vi "addSkipped.vi"(8 "error in (no error)":errorcluster, 10 "test":refnum<class>, 11 "TestResult in":refnum<class "TestResult.lvclass">) -> (0 "error out":errorcluster, 3 "TestResult out":refnum<class "TestResult.lvclass">)   [LabVIEW 2019, in "TestResult.lvclass"]
uses:
  TestResult.lvclass
  resultStatus--enum.ctl
  resultStatusChanged--Cluster.ctl
  TestResult.lvclass/TestResult.ctl
panel:
  # "JKI VI Tester for LabVIEW\nhttp://jkisoft.com/vi-tester\nCopyright (C) 2007-2009, JKI <info@jkisoft.com>\nALL RIGHTS RESERVED"
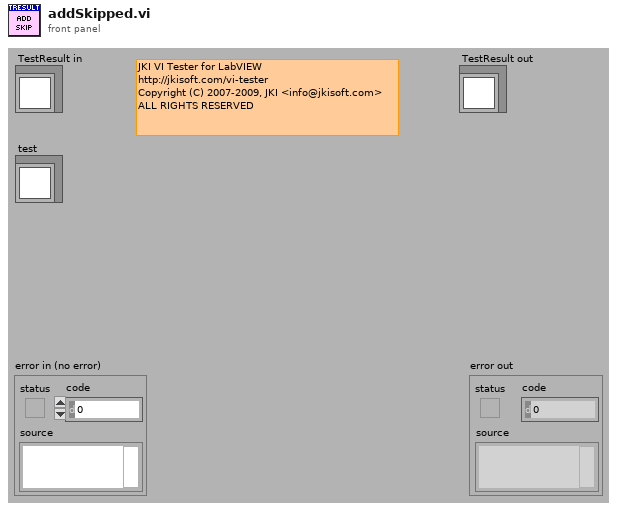
[diagram p1: front panel]
types:
  T1 = typedef "TestResult.lvclass/resultStatusChanged--Cluster.ctl" = cluster{"test":refnum<class>, "resultStatus":T2, "TestResult":refnum<class>, "test error":errorcluster, "execution time (sec)":dbl}
  T2 = typedef "TestResult.lvclass/resultStatus--enum.ctl" = enum16{"testPass", "testFailure", "testError", "testSkipped"}
  T3 = cluster{"test":refnum<class>, "skip error":errorcluster}
  T4 = typedef "TestResult.lvclass/skipped.ctl" = T5[]
  T5 = typedef "TestResult.lvclass/skip.ctl" = cluster{"test":refnum<class>, "error":errorcluster}
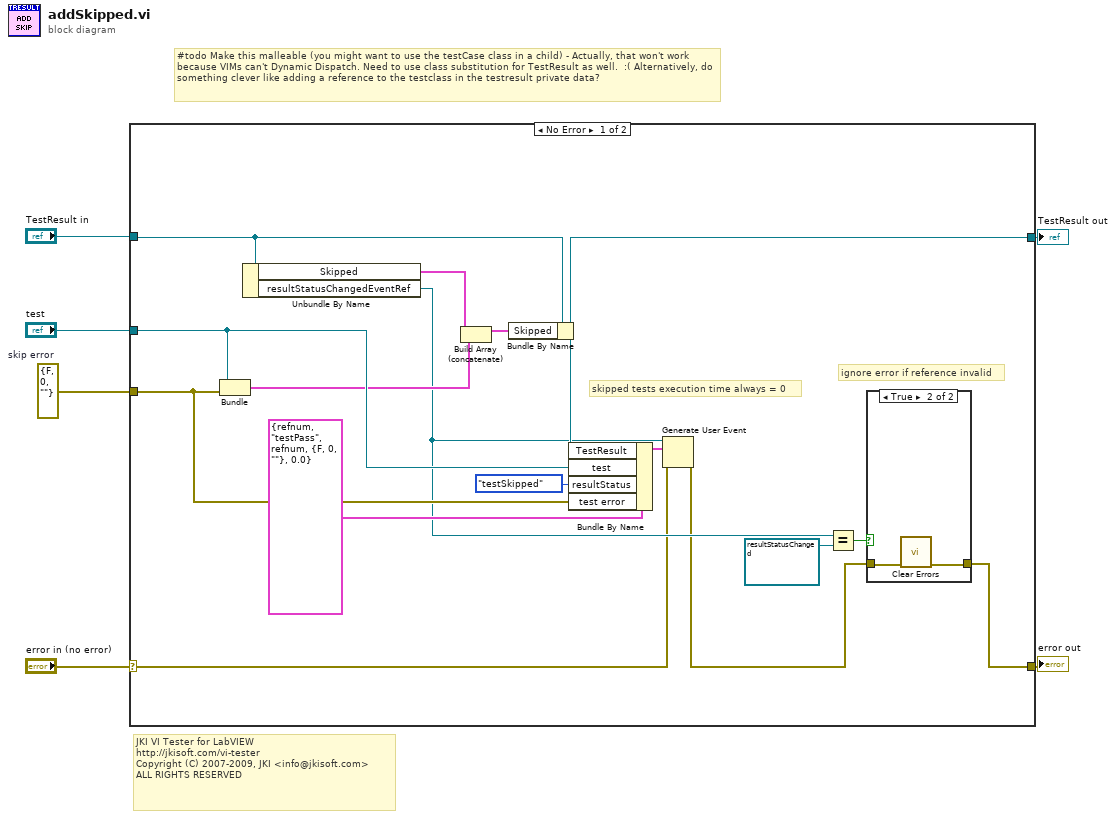
[diagram p0: block diagram]
diagram:
  w1 = errorcluster {"status"=FALSE, "code"=0, "source"=""}  # skip error
  # "#todo Make this malleable (you might want to use the testCase class in a child) - Actually, that won't work because VIMs can't Dynamic Dispatch. Need to use class substitution for TestResult as well.  :( Alternatively, do something clever like adding a reference to the testclass in the testresult private data?"
  # "JKI VI Tester for LabVIEW\nhttp://jkisoft.com/vi-tester\nCopyright (C) 2007-2009, JKI <info@jkisoft.com>\nALL RIGHTS RESERVED"
  n1 = case shown="No Error" "error in (no error)" {
    selector: "error in (no error)" -> [w9 w27]
    tunnel: [w7 w27] -> w5
    tunnel: [w21 w26] -> w3
    tunnel: "TestResult in" -> [w22 w26]
    tunnel: "test" -> [w20 _]
    tunnel: w1 -> [w19 _]
    frame No Error {
      # "skipped tests execution time always = 0"
      # "ignore error if reference invalid"
      n2 = Bundle("test"=w20, "skip error"=w19) -> (w16:T3)  [unwired: 1 in]
      n3 = Unbundle By Name(w22) -> ("Skipped"=w18:T4, "resultStatusChangedEventRef"=w11:refnum<user-event>)
      n4 = Build Array (concatenate)(w18, w16) -> (w17:T4)
      n5 = Bundle By Name(cluster=w22, "Skipped"=w17) -> (w21:refnum<class "TestResult.lvclass">)
      n6 = Bundle By Name(cluster=T1 {"test"=refnum, "resultStatus"=enum."testPass", "TestResult"=refnum, "test error"={"status"=FALSE, "code"=0, "source"=""}, "execution time (sec)"=0.0} ("event data"), "TestResult"=w21, "test"=w20, "resultStatus"=resultStatus--enum."testSkipped", "test error"=w19) -> (w14:T1)
      n7 = Generate User Event(user event=w11, event data cluster=w14, error in=w9) -> (error out=w8:errorcluster)  [unwired: 1 in, 1 out]
      n8 = Equal?(x=w11, y=refnum<user-event> refnum ("resultStatusChangedEventRef")) -> (x = y?=w10:bool)
      n9 = case shown="True" w10 {
        tunnel: [w23 w24] -> w7
        tunnel: w8 -> [w23 w25]
        frame False {
        }
        frame True {
          n10 = call <vilib>:"Clear Errors.vi"("error in (no error)"=w25) -> ("error out"=w24:errorcluster)  [unwired: 5 in, 1 out]
        }
      }
    }
    frame Error {
    }
  }
  "error out" <- w5
  "TestResult out" <- w3
